vi "Application Example 2.vi"() -> ()   [LabVIEW 2025, in "NewtonsPSM1735.lvlib"]
doc: "This Application configure and readback the Scope function of the PPA2530"
uses:
  NewtonsPSM1735.lvlib
panel:
  in  "Pre-Trigger (25%)":u8(slide)=25 max=75 step=25 scale=0.0..75.0
  in  "Trigger HF Reject (Off)":bool
  out "Current Waveform":dbl[][](graph)
  in  "stop":bool
  in  "Trigger  Reference (Voltage)":u16(ring) items=["Voltage", "Current"]
  in  "Trigger Phase (Phase 1)":u16(ring) items=["Phase 1", "Phase 2", "Phase 3"]
  in  "Trigger Type (Auto)":u16(ring) items=["Auto", "Normal", "Single Shot"]
  out "Voltage Waveform":dbl[][](graph)
  out "error out":errorcluster
  in  "VISA resource name":refnum<visa-resource-name>
  in  "Current Ranging Mode (Auto)":u16(ring) items=["AUTO", "UPAUTO", "100 mA", "316 mA", "1 A", "3,16 A", "10 A", "31,6 A", "100 A", "316 A"]
  in  "Voltage Ranging Mode (Auto)":u16(ring) items=["AUTO", "UPAUTO", "1V", "3,16V", "10V", "31,6V", "100V", "316V", "1000V", "3160V"]
  # "PPA2530\nPRECISION  POWER ANALYZER"
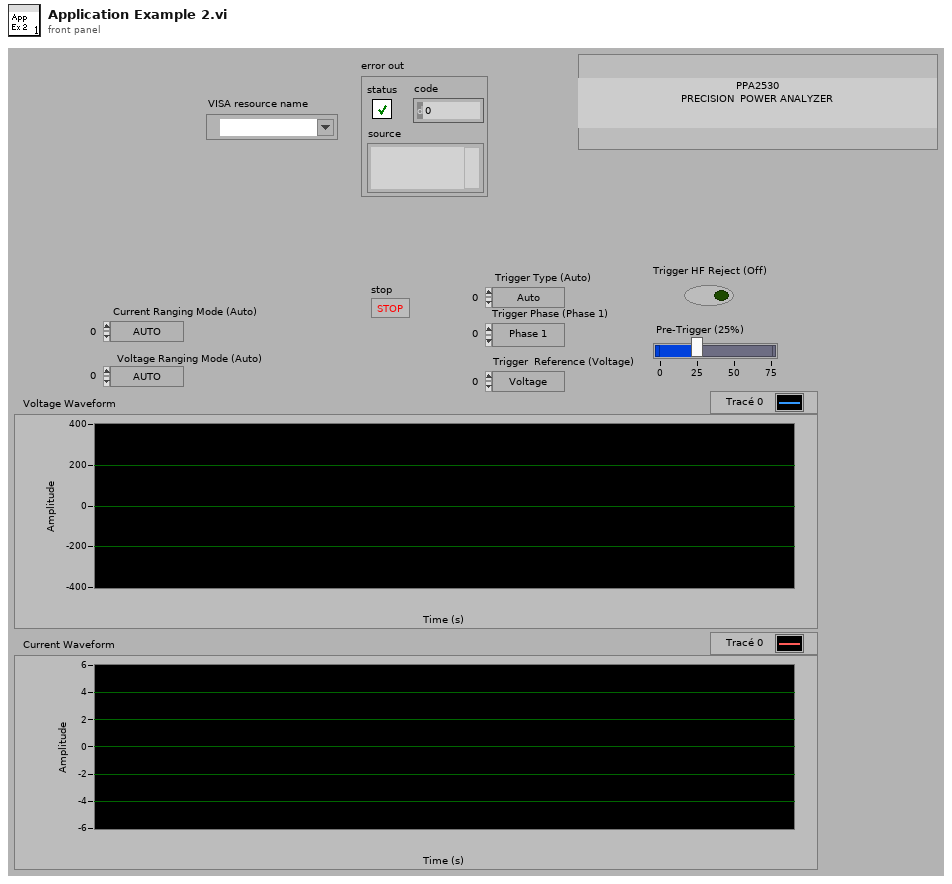
[diagram p1: front panel]
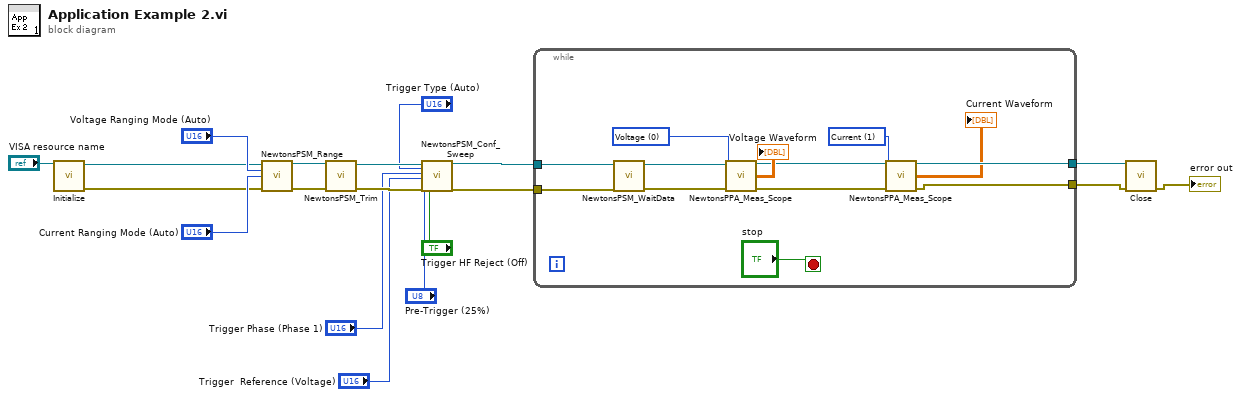
[diagram p0: block diagram]
diagram:
  n1 = call "Initialize.vi"("VISA resource name"="VISA resource name") -> ("error out"=w8:errorcluster, "VISA resource name out"=w9:refnum<visa-resource-name>)  [unwired: 9 in]
  n2 = call "NewtonsPSM_Range.vi"("VISA session"=w9, "Input Ranging Mode (Auto)"="Voltage Ranging Mode (Auto)", "Input Input Type (Internal)"="Current Ranging Mode (Auto)", "error in (no error)"=w8) -> ("dup VISA session"=w18:refnum<visa-resource-name>, "error out"=w19:errorcluster)  [unwired: 10 in]
  n3 = call "NewtonsPSM_Trim.vi"("error in"=w19, "VISA.name"=w18) -> ("error out"=w14:errorcluster, "VISA.name out"=w13:refnum<visa-resource-name>)  [unwired: 8 in]
  n4 = call "NewtonsPSM_Conf_Sweep.vi"("VISA session"=w13, "Steps (Log)"="Trigger Type (Auto)", "Sweep (Single)"="Trigger Phase (Phase 1)", 3:"Trigger  Reference (Voltage)", 4:"Pre-Trigger (25%)", "error in (no error)"=w14, "Frequency Market (Off)"="Trigger HF Reject (Off)") -> ("dup VISA session"=w7:refnum<visa-resource-name>, "error out"=w6:errorcluster)  [unwired: 11 in]
  n5 = while {
    tunnel: w7 -> [w30]
    tunnel: w6 -> [w28]
    tunnel: [w22] -> w4
    tunnel: [w23] -> w3
    stop <- "stop" stop-if-true
    w20 = u16 1 items=["Voltage", "Current"] ("Measurement Type (Voltage)")
    w32 = u16 0 items=["Voltage", "Current"] ("Measurement Type (Voltage)")
    n6 = call "NewtonsPSM_WaitData.vi"("error in (no error)"=w28, "VISA session"=w30) -> ("error out"=w27:errorcluster, "dup VISA session"=w29:refnum<visa-resource-name>)  [unwired: 5 in, 1 out]
    n7 = call "NewtonsPPA_Meas_Scope.vi"("VISA session"=w29, "Measurement Type (Voltage)"=w32, "error in (no error)"=w27) -> ("dup VISA session"=w24:refnum<visa-resource-name>, "Waveform"=→"Voltage Waveform":dbl[][], "error out"=w25:errorcluster)  [unwired: 9 in, 1 out]
    n8 = call "NewtonsPPA_Meas_Scope.vi"("VISA session"=w24, "Measurement Type (Voltage)"=w20, "error in (no error)"=w25) -> ("dup VISA session"=w23:refnum<visa-resource-name>, "Waveform"=→"Current Waveform":dbl[][], "error out"=w22:errorcluster)  [unwired: 9 in, 1 out]
  }
  n9 = call "Close.vi"("error in (no error)"=w4, "VISA resource name"=w3) -> ("error out"=→"error out":errorcluster)  [unwired: 9 in]
